vi "getDescription.vi"(8 "error in (no error)":errorcluster, 11 "Whip in":refnum<class "Whip.lvclass">) -> (0 "error out":errorcluster, 2 "description":string, 3 "Whip out":refnum<class "Whip.lvclass">)   [LabVIEW 2013, in "Whip.lvclass"]
uses:
  Whip.lvclass
  Whip.lvclass/Whip.ctl
  Beverage/Beverage.lvclass
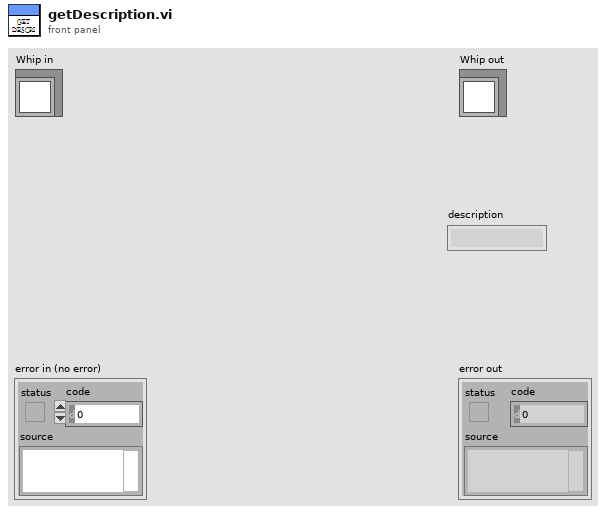
[diagram p1: front panel]
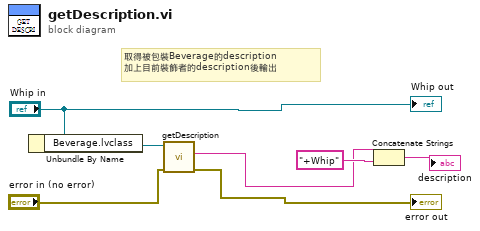
[diagram p0: block diagram]
diagram:
  # "取得被包裝Beverage的description\n加上目前裝飾者的description後輸出"
  n1 = Unbundle By Name("Whip in") -> ("Beverage.lvclass"=w5:refnum<class "Beverage.lvclass">)
  n2 = call-dynamic "getDescription.vi"("error in (no error)"="error in (no error)", "Beverage in"=w5) -> ("error out"=→"error out":errorcluster, "description"=w1:string)  [unwired: 7 in, 1 out]
  n3 = Concatenate Strings(w1, "+Whip" ("description")) -> (→"description":string)
  "Whip out" <- "Whip in"
